vi "GetTrafoParams - Test.vi"() -> ()   [LabVIEW 2017]
uses:
  AT901 API/Structures/Struct TransformationData.ctl
panel:
  in  "TransformationData 2":T1
  out "TransformationData":T1={"dVal1"=0.0, "dVal2"=0.0, "dVal3"=0.0, "dRot1"=0.0, "dRot2"=0.0, "dRot3"=0.0, "dScale"=1.0}
  out "error out":errorcluster
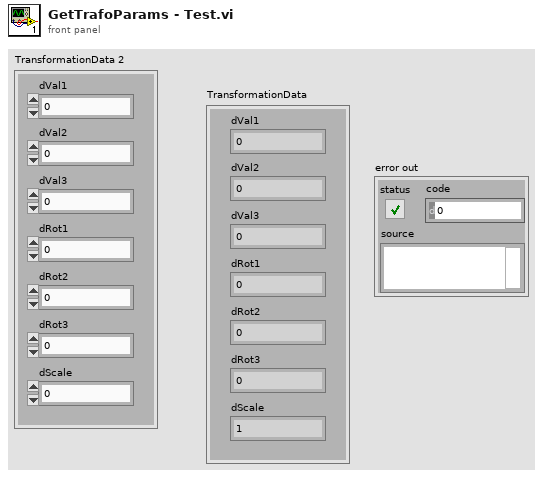
[diagram p1: front panel]
types:
  T1 = typedef "Struct TransformationData.ctl" = cluster{"dVal1":dbl, "dVal2":dbl, "dVal3":dbl, "dRot1":dbl, "dRot2":dbl, "dRot3":dbl, "dScale":dbl}
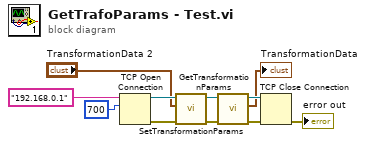
[diagram p0: block diagram]
diagram:
  n1 = TCP Open Connection(address="192.168.0.1", remote port or service name=u16 700) -> (connection ID=w5:refnum<k5>, error out=w2:errorcluster)  [unwired: 3 in]
  n2 = call "SetTransformationParams.vi"("error in (no error)"=w2, "TransformationData"="TransformationData 2", "TCP Network Connection in"=w5) -> ("error out"=w3:errorcluster, "TCP Network Connection out"=w4:refnum<k5>)  [unwired: 5 in, 2 out]
  n3 = call "GetTransformationParams.vi"("error in (no error)"=w3, "TCP Network Connection in"=w4) -> ("error out"=w8:errorcluster, "TransformationData"=→"TransformationData":T1, "TCP Network Connection out"=w7:refnum<k5>)  [unwired: 5 in, 2 out]
  n4 = TCP Close Connection(connection ID=w7, error in (no error)=w8) -> (error out=→"error out":errorcluster)  [unwired: 1 in, 1 out]
